vi "CIRCUITO RC.vi"(4 "C":dbl, 6 "R":dbl, 7 "Array":dbl[](array[numeric]), 9 "t":dbl, 10 "dt":dbl, 11 "t0":dbl) -> (3 "Numeric":dbl)   [LabVIEW 2017]
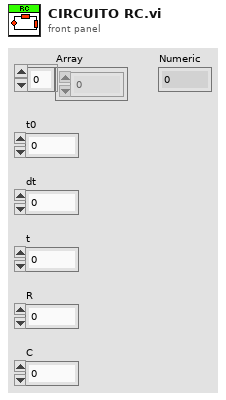
[diagram p1: front panel]
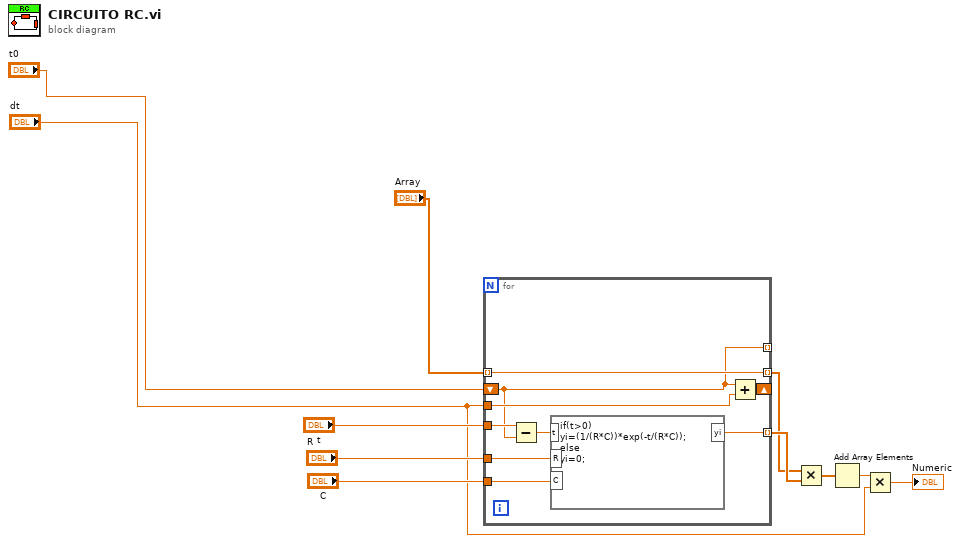
[diagram p0: block diagram]
diagram:
  n1 = for {
    tunnel: "Array" -> [w16] mode=indexing
    shift-right: [w20] -> _
    shift-left: "t0" -> [w12]
    tunnel: "dt" -> [w19]
    tunnel: "R" -> [w15]
    tunnel: "C" -> [w18]
    tunnel: [w17] -> w7 mode=indexing
    tunnel: [w16] -> w6 mode=indexing
    tunnel: "t" -> [w14]
    tunnel: [w12] -> _ mode=indexing
    n2 = Subtract(x=w14, y=w12) -> (x-y=w13:dbl)
    n3 = formula code="if(t>0)\nyi=(1/(R*C))*exp(-t/(R*C));\nelse\nyi=0;"("t"=w13, "R"=w15, "C"=w18) -> ("yi"=w17:dbl)
    n4 = Add(x=w12, y=w19) -> (x+y=w20:dbl)
  }
  n5 = Multiply(x=w6, y=w7) -> (x*y=w8:dbl[])
  n6 = Add Array Elements(numeric array=w8) -> (sum=w9:dbl)
  n7 = Multiply(x=w9, y="dt") -> (x*y=→"Numeric":dbl)
